vi "Sort 1D Array (CDB)__ogtk.vi"(7 "Method (magnitude)":enum16{"real", "imaginary", "magnitude"}(ring)=enum."magnitude", 9 "Order":enum16{"ascending", "descending"}(ring), 11 "Array in":cdb[](array[numeric]) format="%.2f") -> (2 "Sorted Pointers":i32[](array[numeric]), 3 "Sorted Array out":cdb[](array[numeric]) format="%.2f")   [LabVIEW 2014, in "ZLIB.lvlib"]
doc: "This polymorphic VI sorts a 1D array of numerics or strings, regardless of the array size. You can specify whether to sort in ascending or descending order."
uses:
  ZLIB.lvlib
panel:
  # "Sort 1D Array\n\nThis VI sorts a 1D array of any size in descending or ascending order.\n\nPlease visit http://www.OpenG.org to learn about the\nOpen Source LabVIEW software movement.\n\nNOTICE -- YOU MUST LEAVE THIS NOTICE IN PLACE.  PER THE TERMS OF THE LICENSE BELOW, YOU MAY SUBLICENSE THIS SOFTWARE \nIN ANY WAY THAT DOES NOT CONFLICT WITH THIS LICENSE.\n\n### BSD License (http://www.opensource.org/licenses/bsd-license.php) Begin ###\n \nCopyright (c) 2002, Jim Kring <jim@jimkring.com>\nCopyright (c) 2002, Cal-Bay Systems, Inc. <info@calbay.com>\nCopyright (c) 2005, MKS Instruments, Inc., author: Doug Femec<doug_femec@mksinst.com>, IM dafemec\n\nAll rights reserved.\n\nRedistribution and use in source and binary forms, with or without modification, are permitted provided that the following conditions are met:\n\n    * Redistributions of source code must retain the above copyright notice, this list of conditions and the following disclaimer.\n    * Redistributions in binary form must reproduce the above copyright notice, this list of conditions and the following disclaimer in the \n       documentation and/or other materials provided with the distribution.\n    * Neither the name of SciWare, James Kring, Inc., nor the names of its contributors may be used to endorse or promote products derived \n       from this software without specific prior written permission.\n\nTHIS SOFTWARE IS PROVIDED BY THE COPYRIGHT HOLDERS AND CONTRIBUTORS \"AS IS\" AND ANY EXPRESS OR IMPLIED WARRANTIES, \nINCLUDING, BUT NOT LIMITED TO, THE IMPLIED WARRANTIES OF MERCHANTABILITY AND FITNESS FOR A PARTICULAR PURPOSE ARE \nDISCLAIMED. IN NO EVENT SHALL THE COPYRIGHT OWNER OR CONTRIBUTORS BE LIABLE FOR ANY DIRECT, INDIRECT, INCIDENTAL,\n SPECIAL, EXEMPLARY, OR CONSEQUENTIAL DAMAGES (INCLUDING, BUT NOT LIMITED TO, PROCUREMENT OF SUBSTITUTE GOODS OR \nSERVICES; LOSS OF USE, DATA, OR PROFITS; OR BUSINESS INTERRUPTION) HOWEVER CAUSED AND ON ANY THEORY OF LIABILITY, \nWHETHER IN CONTRACT, STRICT LIABILITY, OR TORT (INCLUDING NEGLIGENCE OR OTHERWISE) ARISING IN ANY WAY OUT OF THE USE \nOF THIS SOFTWARE, EVEN IF ADVISED OF THE POSSIBILITY OF SUCH DAMAGE.\n\n### BSD License End ###"
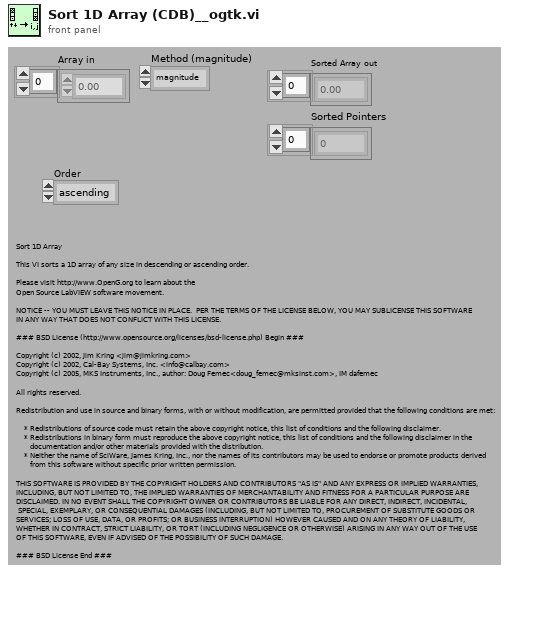
[diagram p1: front panel]
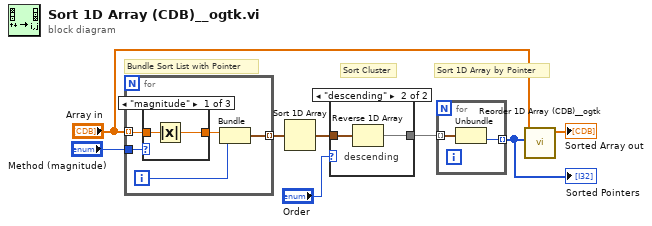
[diagram p0: block diagram]
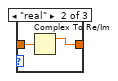
[diagram p2: hidden frame]
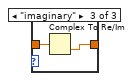
[diagram p3: hidden frame]
diagram:
  # "Sort 1D Array by Pointer"
  # "Sort Cluster"
  # "Bundle Sort List with Pointer"
  n1 = for {
    tunnel: "Array in" -> [w12] mode=indexing
    tunnel: [w13] -> w6 mode=indexing
    tunnel: "Method (magnitude)" -> [w9]
    i -> [w10]
    n2 = case shown="\"magnitude\"" w9 {
      tunnel: w12 -> [w15 w17 w19]
      tunnel: [w14 w16 w18] -> w11
      frame "magnitude" {
        n3 = Absolute Value(x=w15) -> (abs(x)=w14:dbl)
      }
      frame "real" {
        n4 = Complex To Re/Im(x + iy=w17) -> (x=w16:dbl)  [unwired: 1 out]
      }
      frame "imaginary" {
        n5 = Complex To Re/Im(x + iy=w19) -> (y=w18:dbl)  [unwired: 1 out]
      }
    }
    n6 = Bundle(w11, w10) -> (w13:cluster{dbl, i32})  [unwired: 1 in]
  }
  n7 = Sort 1D Array(array=w6) -> (sorted array=w5:cluster{dbl, i32}[])
  n8 = case shown="\"descending\"" "Order" {
    tunnel: [w20 w21] -> w7
    tunnel: w5 -> [w20 w22]
    frame "ascending", Default {
    }
    frame "descending" {
      # "descending"
      n9 = Reverse 1D Array(array=w22) -> (reversed array=w21:cluster{dbl, i32}[])
    }
  }
  n10 = for {
    tunnel: w7 -> [w24] mode=indexing
    tunnel: [w23] -> w1 mode=indexing
    n11 = Unbundle(w24) -> (w23:i32)  [unwired: 1 out]
  }
  "Sorted Pointers" <- w1
  n12 = call "Reorder 1D Array (CDB)__ogtk.vi"("Sorted Pointers in"=w1, "Array in"="Array in") -> ("Sorted Array out"=→"Sorted Array out":cdb[])  [unwired: 8 in, 1 out]
